vi "SwerveDriveControl.vi"(9 "Swerve Drive Param":T1(ring), 10 "Inputs":dbl[](array[numeric])) -> (2 "Speed":dbl)   [LabVIEW 2016]
uses:
  Robot Global Data.vi
  <vilib>/Rock Robotics/Network Tables/NT Write Number.vi
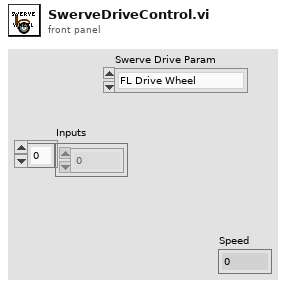
[diagram p1: front panel]
types:
  T1 = enum16{"FL Drive Wheel", "FR Drive Wheel", "RL Drive Wheel", "RR Drive Wheel", "FL Steer Wheel", "FR Steer Wheel", "RL Steer Wheel", "RR Steer Wheel"}
  T2 = enum16{"Z", "Y", "X", "Rot. Point X", "Rot. Point Y", "Width/2", "Max", "Length/2"}
  T3 = enum16{"Z Axis", "Y", "X", "Rot. Point X", "Rot. Point Y", "Width/2", "Max", "Length/2"}
  T4 = enum16{"min count rotation", "max count rotation ", "offset count to zero wheel"}
  T5 = enum16{"Sensor Position", "Sensor Velocity", "Rotations", "Angle"}
  T6 = typedef "WPI_MotorControlDeviceRef.ctl" = cluster{"DeviceStatus":errorcluster, "Type":T7, "PWM":cluster{"PWM Channel":T8, "DeadBand":T9}, "CAN":cluster{"Device Number":u8, "SetOutput VI Ref":variant, "GetOutput VI Ref":variant, "Enable VI Ref":variant, "Disable VI Ref":variant, "Data":variant}, "Invert":bool}
  T7 = typedef "WPI_MotorControlType.ctl" = enum16{"PWM", "CAN"}
  T8 = typedef "FPGA_DIOPWMChannel.ctl" = enum8{"PWM 0", "PWM 1", "PWM 2", "PWM 3", "PWM 4", "PWM 5", "PWM 6", "PWM 7", "PWM 8", "PWM 9", "PWM MXP 0", "PWM MXP 1", "PWM MXP 2", "PWM MXP 3", "PWM MXP 4", "PWM MXP 5", "PWM MXP 6", "PWM MXP 7", "PWM MXP 8", "PWM MXP 9", "Invalid"}
  T9 = typedef "WPI_PWMDeadband.ctl" = cluster{"Name":string, "maxPositivePwm":i32, "minPositivePwm":i32, "centerPwm":i32, "maxNegativePwm":i32, "minNegativePwm":i32, "angularRange":u16}
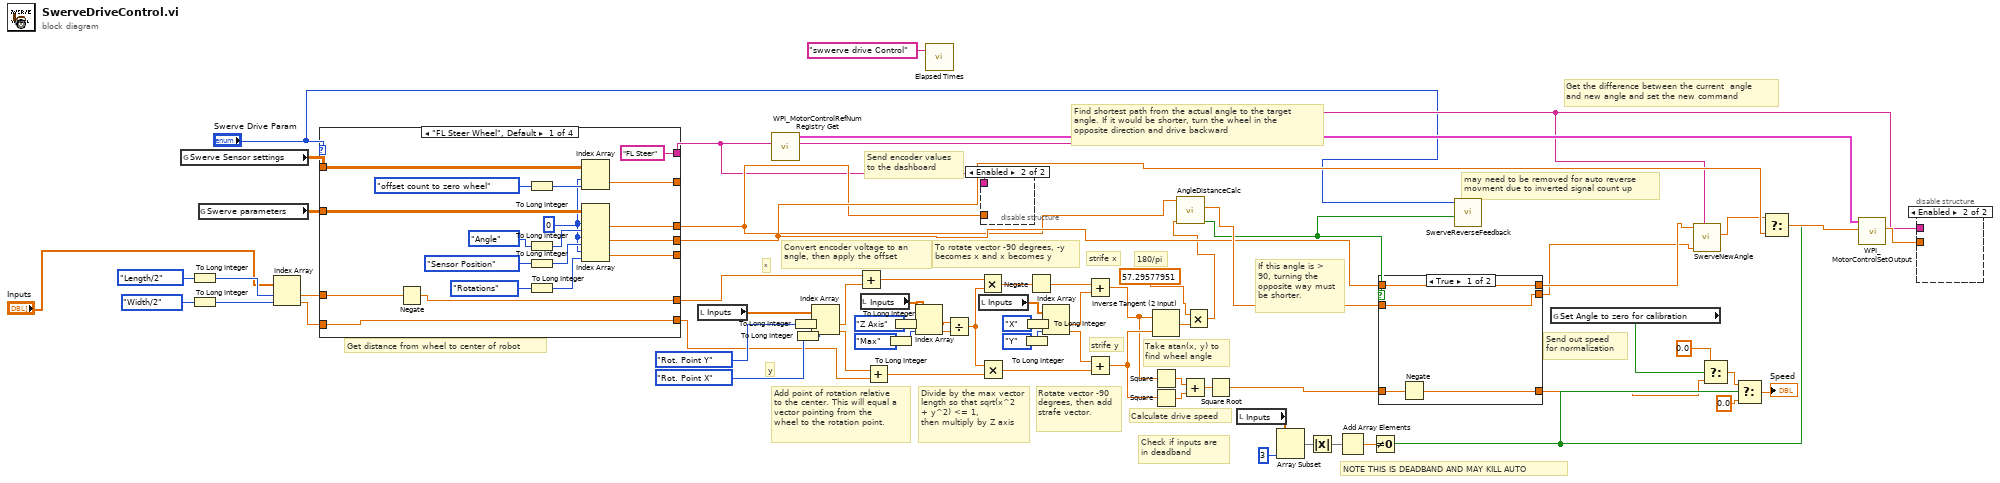
[diagram p0: block diagram]
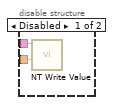
[diagram p2: hidden frame]
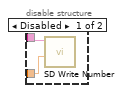
[diagram p3: hidden frame]
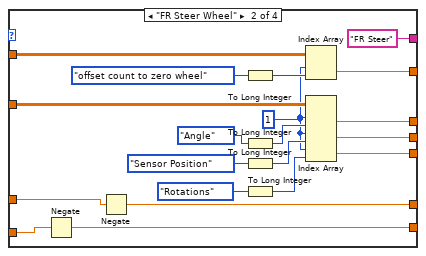
[diagram p5: hidden frame]
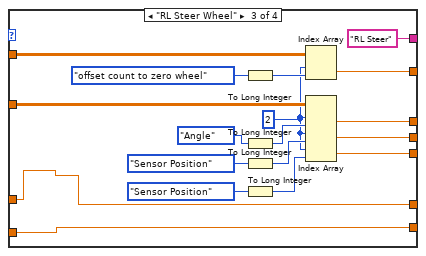
[diagram p6: hidden frame]
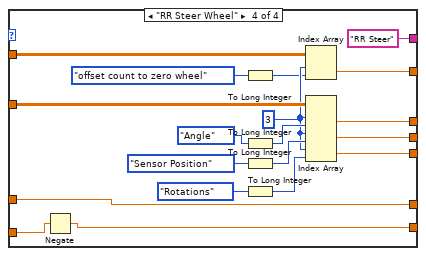
[diagram p7: hidden frame]
diagram:
  # "may need to be removed for auto reverse\nmovment due to inverted signal count up"
  # "NOTE THIS IS DEADBAND AND MAY KILL AUTO"
  # "strife x"
  # "strife y"
  # "x"
  # "y"
  # "180/pi"
  # "Send out speed\nfor normalization"
  # "Get the difference between the current  angle\nand new angle and set the new command"
  # "Send encoder values \nto the dashboard"
  # "To rotate vector -90 degrees, -y becomes x and x becomes y"
  # "Divide by the max vector length so that sqrt(x^2 + y^2) <= 1,\nthen multiply by Z axis"
  # "Add point of rotation relative to the center. This will equal a vector pointing from the\nwheel to the rotation point."
  # "Check if inputs are\nin deadband"
  # "Convert encoder voltage to an angle, then apply the offset"
  # "If this angle is > 90, turning the opposite way must be shorter."
  # "Find shortest path from the actual angle to the target angle. If it would be shorter, turn the wheel in the opposite direction and drive backward"
  # "Take atan(x, y) to find wheel angle"
  # "Calculate drive speed"
  # "Rotate vector -90 degrees, then add strafe vector."
  # "Get distance from wheel to center of robot"
  n1 = global read "Robot Global Data.vi" "Swerve Sensor settings"() -> (w16:dbl[][])
  n2 = To Long Integer(number=T2."Length/2") -> (32bit integer=w31:i32)
  n3 = To Long Integer(number=T2."Width/2") -> (32bit integer=w30:i32)
  n4 = global read "Robot Global Data.vi" "Swerve parameters"() -> (w40:dbl[][])
  n5 = Index Array(array="Inputs", index #1=w31, index #2=w30) -> (element #1=w37:dbl, element #2=w32:dbl)
  n6 = case shown="\"FL Steer Wheel\", Default" "Swerve Drive Param" {
    tunnel: ["FL Steer" "FR Steer" "RL Steer" "RR Steer"] -> w11
    tunnel: [w74 w107 w113 w132] -> w34
    tunnel: w40 -> [w91 w111 w129 w148]
    tunnel: w37 -> [w88 w92 w113 w132]
    tunnel: [w73 w108 w112 w131] -> w35
    tunnel: [w86 w105 w125 w144] -> w23
    tunnel: [w83 w102 w122 w141] -> w33
    tunnel: w32 -> [w73 w101 w112 w130]
    tunnel: [w80 w99 w120 w139] -> _
    tunnel: w16 -> [w76 w95 w116 w134]
    tunnel: [w75 w93 w114 w133] -> _
    frame "FL Steer Wheel", Default {
      w77 = 0 ("disabled index (row)")
      n7 = Negate(x=w88) -> (-x=w74:dbl)
      n8 = To Long Integer(number=T4."offset count to zero wheel" ("SwerveSensorSetting")) -> (32bit integer=w78:i32)
      n9 = To Long Integer(number=T5."Angle" ("Swerve Parameters def")) -> (32bit integer=w89:i32)
      n10 = To Long Integer(number=T5."Sensor Position" ("Swerve Parameters def")) -> (32bit integer=w84:i32)
      n11 = To Long Integer(number=T5."Rotations" ("Swerve Parameters def")) -> (32bit integer=w81:i32)
      n12 = Index Array(array=w76, index (row)=w77, index (col)=w78) -> (element=w75:dbl)
      n13 = Index Array(array=w91, index (row) #1=w77, index (col) #1=w89, index (row) #2=w77, index (col) #2=w84, index (row) #3=w77, index (col) #3=w81) -> (element #1=w86:dbl, element #2=w83:dbl, element #3=w80:dbl)
    }
    frame "FR Steer Wheel" {
      w94 = 1 ("disabled index (row)")
      n14 = Negate(x=w101) -> (-x=w108:dbl)
      n15 = Negate(x=w92) -> (-x=w107:dbl)
      n16 = To Long Integer(number=T4."offset count to zero wheel" ("SwerveSensorSetting")) -> (32bit integer=w96:i32)
      n17 = To Long Integer(number=T5."Angle" ("Swerve Parameters def")) -> (32bit integer=w109:i32)
      n18 = To Long Integer(number=T5."Sensor Position" ("Swerve Parameters def")) -> (32bit integer=w103:i32)
      n19 = To Long Integer(number=T5."Rotations" ("Swerve Parameters def")) -> (32bit integer=w98:i32)
      n20 = Index Array(array=w95, index (row)=w94, index (col)=w96) -> (element=w93:dbl)
      n21 = Index Array(array=w111, index (row) #1=w94, index (col) #1=w109, index (row) #2=w94, index (col) #2=w103, index (row) #3=w94, index (col) #3=w98) -> (element #1=w105:dbl, element #2=w102:dbl, element #3=w99:dbl)
    }
    frame "RL Steer Wheel" {
      w115 = 2 ("disabled index (row)")
      n22 = To Long Integer(number=T4."offset count to zero wheel" ("SwerveSensorSetting")) -> (32bit integer=w117:i32)
      n23 = To Long Integer(number=T5."Angle" ("Swerve Parameters def")) -> (32bit integer=w127:i32)
      n24 = To Long Integer(number=T5."Sensor Position" ("Swerve Parameters def")) -> (32bit integer=w123:i32)
      n25 = To Long Integer(number=T5."Sensor Position" ("Swerve Parameters def")) -> (32bit integer=w119:i32)
      n26 = Index Array(array=w116, index (row)=w115, index (col)=w117) -> (element=w114:dbl)
      n27 = Index Array(array=w129, index (row) #1=w115, index (col) #1=w127, index (row) #2=w115, index (col) #2=w123, index (row) #3=w115, index (col) #3=w119) -> (element #1=w125:dbl, element #2=w122:dbl, element #3=w120:dbl)
    }
    frame "RR Steer Wheel" {
      w137 = 3 ("disabled index (row)")
      n28 = Negate(x=w130) -> (-x=w131:dbl)
      n29 = To Long Integer(number=T4."offset count to zero wheel" ("SwerveSensorSetting")) -> (32bit integer=w135:i32)
      n30 = To Long Integer(number=T5."Angle" ("Swerve Parameters def")) -> (32bit integer=w146:i32)
      n31 = To Long Integer(number=T5."Sensor Position" ("Swerve Parameters def")) -> (32bit integer=w142:i32)
      n32 = To Long Integer(number=T5."Rotations" ("Swerve Parameters def")) -> (32bit integer=w138:i32)
      n33 = Index Array(array=w134, index (row)=w137, index (col)=w135) -> (element=w133:dbl)
      n34 = Index Array(array=w148, index (row) #1=w137, index (col) #1=w146, index (row) #2=w137, index (col) #2=w142, index (row) #3=w137, index (col) #3=w138) -> (element #1=w144:dbl, element #2=w141:dbl, element #3=w139:dbl)
    }
  }
  n35 = local read "Inputs"() -> (w22:dbl[])
  n36 = call <vilib>:"WPI_MotorControlRefNum Registry Get.vi"("refnum name"=w11) -> ("MotorControlDevRef"=w12:T6)  [unwired: 9 in, 1 out]
  n37 = To Long Integer(number=T2."Rot. Point Y") -> (32bit integer=w29:i32)
  n38 = To Long Integer(number=T2."Rot. Point X") -> (32bit integer=w28:i32)
  n39 = Index Array(array=w22, index #1=w29, index #2=w28) -> (element #1=w58:dbl, element #2=w59:dbl)
  n40 = Add(x=w34, y=w58) -> (x+y=w41:dbl)
  n41 = local read "Inputs"() -> (w20:dbl[])
  n42 = Add(x=w59, y=w35) -> (x+y=w53:dbl)
  n43 = To Long Integer(number=T2."Max") -> (32bit integer=w26:i32)
  n44 = To Long Integer(number=T3."Z Axis") -> (32bit integer=w27:i32)
  n45 = Index Array(array=w20, index #1=w27, index #2=w26) -> (element #1=w54:dbl, element #2=w55:dbl)
  n46 = call "Elapsed Times.vi"("Call Name"="swwerve drive Control") -> ()  [unwired: 2 in, 1 out]
  n47 = Divide(x=w54, y=w55) -> (x/y=w52:dbl)
  n48 = Multiply(x=w41, y=w52) -> (x*y=w43:dbl)
  n49 = local read "Inputs"() -> (w21:dbl[])
  n50 = Multiply(x=w52, y=w53) -> (x*y=w48:dbl)
  n51 = disable-structure shown="Enabled" {
    disable-tunnel: w23 -> [w150 _]
    disable-tunnel: w11 -> [w149 _]
    frame Disabled {
      n52 = call <vilib>:"SD Write Number.vi"("Numeric"=w150, "Name"=w149) -> ()  [unwired: 8 in, 2 out]
    }
    frame Enabled {
    }
  }
  n53 = To Long Integer(number=T2."Y") -> (32bit integer=w24:i32)
  n54 = To Long Integer(number=T2."X") -> (32bit integer=w25:i32)
  n55 = Negate(x=w43) -> (-x=w42:dbl)
  n56 = Index Array(array=w21, index #1=w25, index #2=w24) -> (element #1=w46:dbl, element #2=w47:dbl)
  n57 = Add(x=w42, y=w46) -> (x+y=w44:dbl)
  n58 = Add(x=w47, y=w48) -> (x+y=w45:dbl)
  n59 = Inverse Tangent (2 Input)(1:w45, 2:w44) -> (0:w18:dbl)
  n60 = Square(x=w44) -> (x^2=w49:dbl)
  n61 = Square(x=w45) -> (x^2=w70:dbl)
  n62 = Add(x=w49, y=w70) -> (x+y=w69:dbl)
  n63 = Multiply(x=57.29577951, y=w18) -> (x*y=w10:dbl)
  n64 = call "AngleDistanceCalc.vi"("Target Angle"=w10, "Current Angle"=w23) -> ("Invert drive"=w6:bool, "Angle Distance"=w36:dbl)  [unwired: 8 in]
  n65 = Square Root(x=w69) -> (sqrt(x)=w68:dbl)
  n66 = local read "Inputs"() -> (w7:dbl[])
  n67 = Array Subset(array=w7, length=3) -> (w66:dbl[])  [unwired: 1 in]
  n68 = Absolute Value(x=w66) -> (abs(x)=w62:dbl[])
  n69 = Add Array Elements(numeric array=w62) -> (sum=w71:dbl)
  n70 = Not Equal To 0?(x=w71) -> (x != 0?=w63:bool)
  n71 = case shown="True" w6 {
    tunnel: w36 -> [w151 w155]
    tunnel: [w153 w157] -> w4
    tunnel: w68 -> [w154 w157]
    tunnel: [w151 w155] -> w14
    tunnel: [w152 w156] -> w15
    tunnel: w33 -> [w152 w156]
    frame True {
      n72 = Negate(x=w154) -> (-x=w153:dbl)
    }
    frame False {
    }
  }
  n73 = call "SwerveReverseFeedback.vi"("Invert Feedback Sensor"=w6, "Swerve Drive Param"="Swerve Drive Param") -> ()  [unwired: 10 in]
  n74 = global read "Robot Global Data.vi" "Set Angle to zero for calibration"() -> (w3:bool)
  n75 = call "SwerveNewAngle.vi"("String"=w11, "Request Angle"=w14, "Current Position"=w15) -> ("Set Position"=w13:dbl)  [unwired: 7 in]
  n76 = Select(t=0.0, s=w3, f=w4) -> (s? t:f=w5:dbl)
  n77 = Select(t=w5, s=w63, f=0.0) -> (s? t:f=→"Speed":dbl)
  n78 = Select(t=w13, s=w63, f=w33) -> (s? t:f=w67:dbl)
  n79 = call <vilib>:"WPI_MotorControlSetOutput.vi"("Output"=w67, "MotorControlDevRef"=w12) -> ("Motor Output"=w19:dbl)  [unwired: 7 in, 2 out]
  n80 = disable-structure shown="Enabled" {
    disable-tunnel: w19 -> [w159 _]
    disable-tunnel: w11 -> [w158 _]
    frame Disabled {
      n81 = call-poly <vilib>:"NT Write Value.vi"("Numeric"=w159, "Name"=w158) -> ()  [unwired: 9 in, 1 out]
    }
    frame Enabled {
    }
  }
